vi "Build Attribute ID.vi"(10 "Attr Name":string, 11 "Unique ID":string) -> (3 "Attr ID Out":string)   [LabVIEW 2019, in "Linked Lists.lvlib" / "Linked List.lvclass"]
uses:
  <vilib>/gpm_packages/@cs/linked-list/Source/Linked List/Linked List/Linked List.lvclass
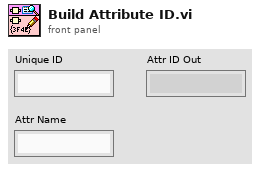
[diagram p1: front panel]
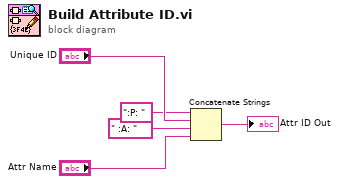
[diagram p0: block diagram]
diagram:
  n1 = Concatenate Strings(":P: " ("string"), "Unique ID", " :A: " ("string"), "Attr Name") -> (→"Attr ID Out":string)
